vi "汇总各次拍照结果存档.vi"(8 "ModelEditInfo":T1={"Root"=path "", "AllModelFold"=path "", "AllModelNamePath"=path "", "所有零件型号"=[], "当前零件型号"="", "所有建立零件信息"=[], "当前零件序号"=0, "当前产品所有点位信息"={"当前点位序号"=0, "点位信息路径"=path "", "CAD点位坐标路径"=path "", "点位信息表"=[], "当前点位信息"={"点位名称"="", "点位坐标(图纸)"={"X"=0.0, "Y"=0.0, "Z"=0.0}, "点位坐标(实际)"={"X"=0.0, "Y"=0.0, "Z"=0.0, "R"=0.0}, "补偿值"={"X"=0.0, "Y"=0.0, "Z"=0.0}, "锁附时机械手角度"=enum."0度", "放料点相对于Mark\n拍照点高度差"=0.0, "选择螺丝托盘"=enum."托盘1", "拧紧程式序号"=0, "自动锁螺丝"=FALSE}, "CAD图纸点位个数"=0}, "当前产品信息"={"产品型号"="J016-9STWH-A插头", "螺丝刀型号"=enum."螺丝刀5-2.5*4mm", "载具上放几片PCB"=0, "1片PCB锁几颗螺丝"=0, "CAD点位坐标文档路径"=path "", "托盘1螺丝型号"=enum."十字螺丝M5*12", "托盘2螺丝型号"=enum."十字螺丝M5*12", "托盘3螺丝型号"=enum."不供料", "托盘4螺丝型号"=enum."不供料", "托盘5螺丝型号"=enum."一字螺丝M2.5*8", "托盘6螺丝型号"=enum."一字螺丝M2.5*8", "托盘7螺丝型号"=enum."一字螺丝M2.5*8", "托盘8螺丝型号"=enum."一字螺丝M2.5*8", "托盘1螺丝锁紧程式序号"=1, "托盘2螺丝锁紧程式序号"=0, "托盘3螺丝锁紧程式序号"=0, "托盘4螺丝锁紧程式序号"=0, "托盘5螺丝锁紧程式序号"=0, "托盘6螺丝锁紧程式序号"=0, "托盘7螺丝锁紧程式序号"=0, "托盘8螺丝锁紧程式序号"=0, "预锁程式序号"=0, "复锁程式序号"=0, "上相机拍PCB孔曝光时间"=0, "上相机取料拍螺帽曝光时间"=0, "上相机复锁拍螺帽曝光时间"=0, "下相机曝光时间"=0}, "所有螺丝和垫片型号"=[], "所有螺丝和垫片型号Path"=path "", "Mark拍照点坐标"=[], "自动锁螺丝: PCB孔拍照点坐标-多片PCB(去除未勾选的)"=[], "8个供料盘是否供料-1PCB(去除未勾选的)"=[], "8个供料盘是否拍照取料"=[], "自动锁螺丝: 1PCB每颗螺丝来自哪个供料盘U8(去除未勾选的)"=[], "自动锁螺丝: 1PCB每颗螺丝拧紧程式编号U8(去除未勾选的)"=[], "4个预锁程式+4个复锁程式编号U8"=[], "自动锁螺丝: 锁螺丝相对拍照时旋转角度-多片PCB(去除未勾选的)"=[], "自动锁螺丝: 点位补偿值-多片PCB(去除未勾选的)"=[], "1PCB上自动锁螺丝个数(去除未勾选的)"=0, "自动锁螺丝: 放料点相对拍照点高度差-多片PCB(去除未勾选的)"=[], "8个供料盘是否供料(包括未勾选的)"=[], "已勾选的自动锁螺丝点位供料盘设定错误"=FALSE} {"当前产品信息"."载具上放几片PCB" min=1 max=4; "当前产品信息"."托盘8螺丝锁紧程式序号" min=1 max=150 step=1; "当前产品信息"."托盘7螺丝锁紧程式序号" min=1 max=150 step=1; "当前产品信息"."托盘6螺丝锁紧程式序号" min=1 max=150 step=1; "当前产品信息"."托盘5螺丝锁紧程式序号" min=1 max=150 step=1; "当前产品信息"."复锁程式序号" min=1 max=150 step=1; "当前产品信息"."预锁程式序号" min=1 max=150 step=1; "当前产品信息"."托盘4螺丝锁紧程式序号" min=1 max=150 step=1; "当前产品信息"."托盘3螺丝锁紧程式序号" min=1 max=150 step=1; "当前产品信息"."托盘2螺丝锁紧程式序号" min=1 max=150 step=1; "当前产品信息"."托盘1螺丝锁紧程式序号" min=1 max=150 step=1; "当前产品所有点位信息"."当前点位信息"."放料点相对于Mark\n拍照点高度差" format="%.3g"}, 9 "不同产品总结果":bool[](array[boolean]), 11 "缓存待存储数据输入":T10) -> (0 "每个数据结果":bool[][](array[boolean]), 1 "数据":string[][](array[string]), 3 "存档数据为空":bool)   [LabVIEW 2014]
uses:
  ModelEditSubVIs/ModeEditeControl.ctl
  Controls/XYZPos.ctl
  Controls/XYZRPos.ctl
  ModelEditSubVIs/ModelInfo.ctl
  Global.vi
panel:
  out "波形图 2":dbl[][](graph)
  out "波形图":dbl[][](graph)
  # "mm   往下为正"
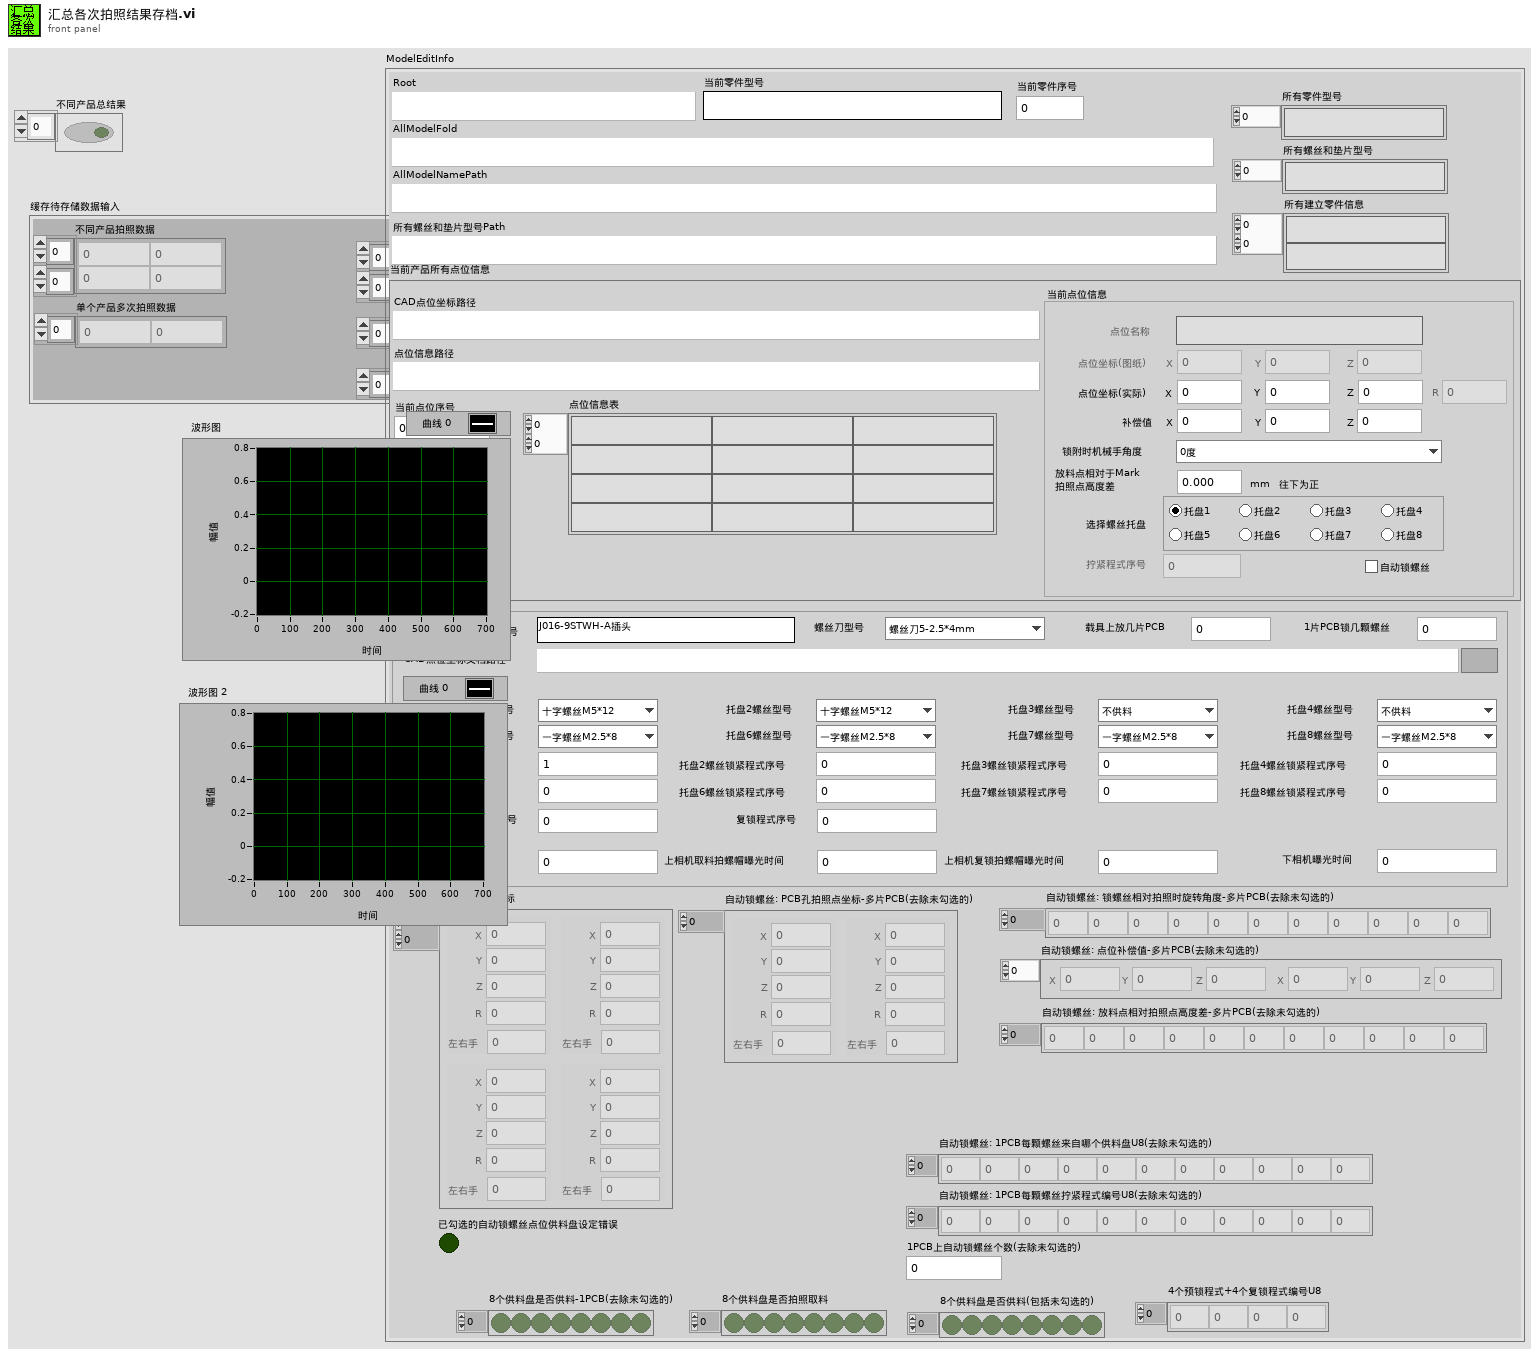
[diagram p1: front panel]
types:
  T1 = typedef "ModeEditeControl.ctl" = cluster{"Root":path, "AllModelFold":path, "AllModelNamePath":path, "所有零件型号":string[], "当前零件型号":string, "所有建立零件信息":string[][], "当前零件序号":i32, "当前产品所有点位信息":cluster{"当前点位序号":i32, "点位信息路径":path, "CAD点位坐标路径":path, "点位信息表":string[][], "当前点位信息":T2, "CAD图纸点位个数":i32}, "当前产品信息":T6, "所有螺丝和垫片型号":string[], "所有螺丝和垫片型号Path":path, "Mark拍照点坐标":T9[][], "自动锁螺丝: PCB孔拍照点坐标-多片PCB(去除未勾选的)":T9[], "8个供料盘是否供料-1PCB(去除未勾选的)":bool[], "8个供料盘是否拍照取料":bool[], "自动锁螺丝: 1PCB每颗螺丝来自哪个供料盘U8(去除未勾选的)":u8[], "自动锁螺丝: 1PCB每颗螺丝拧紧程式编号U8(去除未勾选的)":u8[], "4个预锁程式+4个复锁程式编号U8":u8[], "自动锁螺丝: 锁螺丝相对拍照时旋转角度-多片PCB(去除未勾选的)":i32[], "自动锁螺丝: 点位补偿值-多片PCB(去除未勾选的)":T3[], "1PCB上自动锁螺丝个数(去除未勾选的)":i32, "自动锁螺丝: 放料点相对拍照点高度差-多片PCB(去除未勾选的)":dbl[], "8个供料盘是否供料(包括未勾选的)":bool[], "已勾选的自动锁螺丝点位供料盘设定错误":bool}
  T2 = typedef "锁附点位信息.ctl" = cluster{"点位名称":string, "点位坐标(图纸)":T3, "点位坐标(实际)":T4, "补偿值":T3, "锁附时机械手角度":T5, "放料点相对于Mark\n拍照点高度差":dbl, "选择螺丝托盘":enum32{"托盘1", "托盘2", "托盘3", "托盘4", "托盘5", "托盘6", "托盘7", "托盘8"}, "拧紧程式序号":u16, "自动锁螺丝":bool}
  T3 = typedef "XYZPos.ctl" = cluster{"X":dbl, "Y":dbl, "Z":dbl}
  T4 = typedef "XYZRPos.ctl" = cluster{"X":dbl, "Y":dbl, "Z":dbl, "R":dbl}
  T5 = typedef "锁附时机械手角度.ctl" = enum16{"0度", "顺时针90度", "顺时针180度", "逆时针90度", "逆时针180度"}
  T6 = typedef "ModelInfo.ctl" = cluster{"产品型号":string, "螺丝刀型号":T7, "载具上放几片PCB":u16, "1片PCB锁几颗螺丝":u16, "CAD点位坐标文档路径":path, "托盘1螺丝型号":T8, "托盘2螺丝型号":T8, "托盘3螺丝型号":T8, "托盘4螺丝型号":T8, "托盘5螺丝型号":T8, "托盘6螺丝型号":T8, "托盘7螺丝型号":T8, "托盘8螺丝型号":T8, "托盘1螺丝锁紧程式序号":u32, "托盘2螺丝锁紧程式序号":u32, "托盘3螺丝锁紧程式序号":u32, "托盘4螺丝锁紧程式序号":u32, "托盘5螺丝锁紧程式序号":u32, "托盘6螺丝锁紧程式序号":u32, "托盘7螺丝锁紧程式序号":u32, "托盘8螺丝锁紧程式序号":u32, "预锁程式序号":u32, "复锁程式序号":u32, "上相机拍PCB孔曝光时间":u32, "上相机取料拍螺帽曝光时间":u32, "上相机复锁拍螺帽曝光时间":u32, "下相机曝光时间":u32}
  T7 = typedef "螺丝刀类型.ctl" = enum16{"螺丝刀1-1*3mm", "螺丝刀2-1.5*3mm", "螺丝刀3-2*3mm", "螺丝刀4-2*4mm", "螺丝刀5-2.5*4mm"}
  T8 = typedef "控件-螺丝型号.ctl" = enum16{"不供料", "一字螺丝M2.5*8", "一字螺丝M3*10", "一字螺丝M5*8", "一字螺丝M5*12", "十字螺丝M3*8", "十字螺丝M3*12", "十字螺丝M5*8", "十字螺丝M5*12"}
  T9 = typedef "XYZRPos+左右手.ctl" = cluster{"坐标":T4, "左右手":dbl}
  T10 = typedef "控件-缓存数据.ctl" = cluster{"不同产品拍照数据":dbl[][], "不同产品拍照结果":bool[][], "单个产品多次拍照数据":dbl[], "单个产品多次拍照结果":bool[], "不同产品总结果":bool[]}
  T11 = cluster{"不同产品拍照数据":dbl[], "不同产品拍照结果":bool[], "布尔":bool, bool}
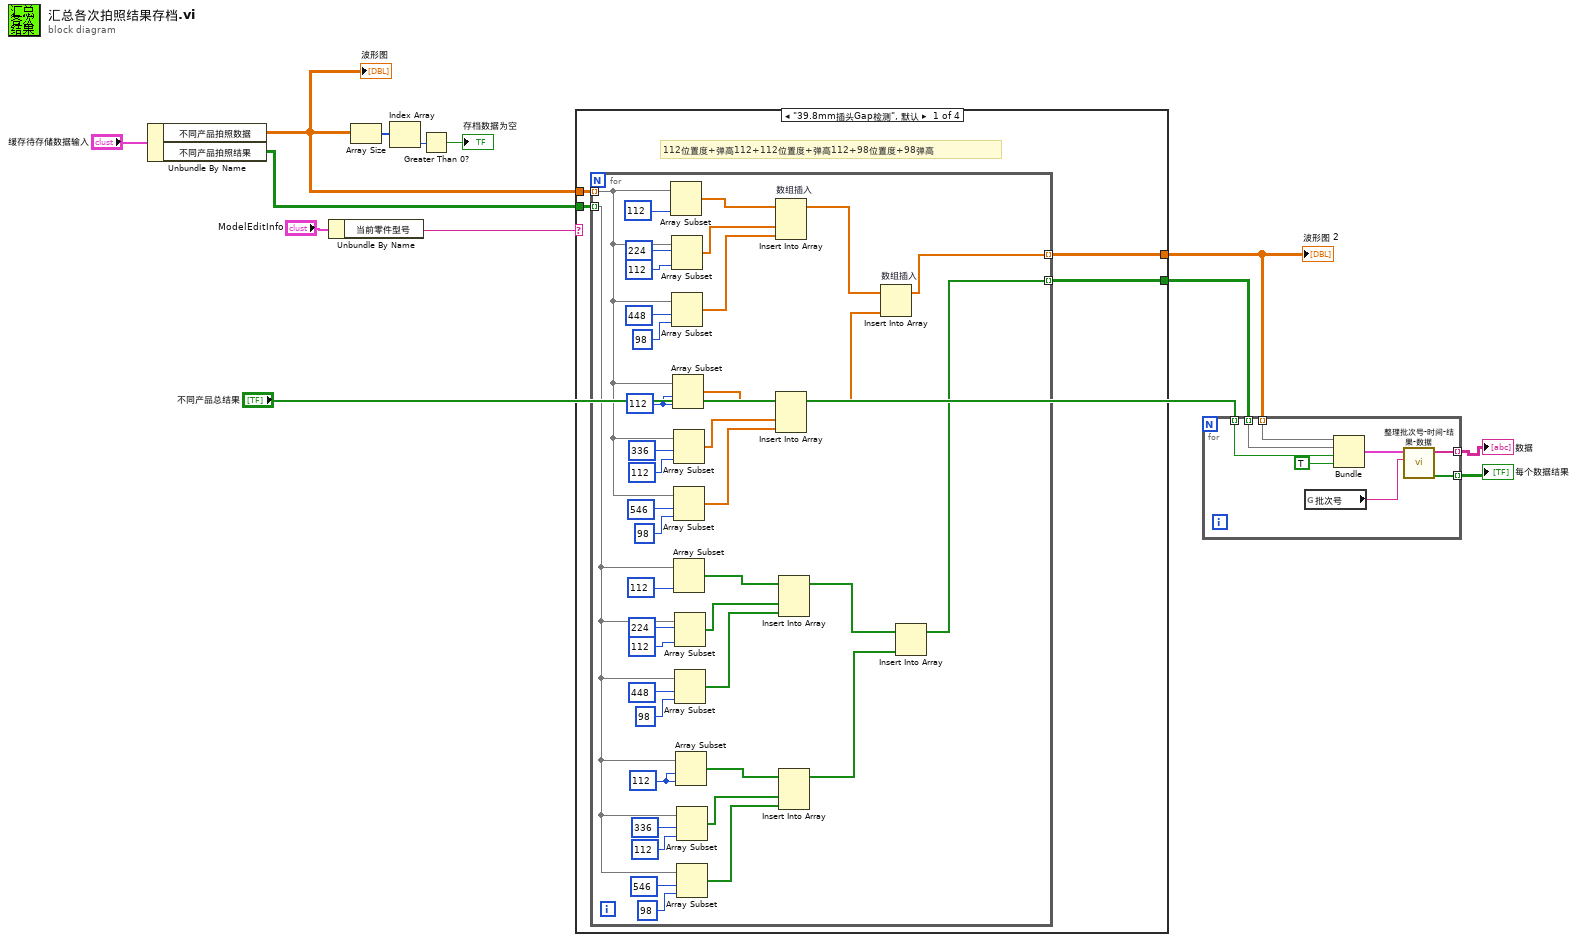
[diagram p0: block diagram]
diagram:
  n1 = Unbundle By Name("缓存待存储数据输入") -> ("不同产品拍照数据"=w6:dbl[][], "不同产品拍照结果"=w5:bool[][])
  "波形图" <- w6
  n2 = Unbundle By Name("ModelEditInfo") -> ("当前零件型号"=w8:string)
  n3 = Array Size(array=w6) -> (size(s)=w11:i32[])
  n4 = Index Array(array=w11) -> (element=w12:i32)  [unwired: 1 in]
  n5 = Greater Than 0?(x=w12) -> (x > 0?=→"存档数据为空":bool)
  n6 = case shown="\"39.8mm插头Gap检测\", 默认" w8 {
    tunnel: w6 -> [w17 w59 w61 w63]
    tunnel: w5 -> [w16 w58 w60 w62]
    tunnel: [w14 w59 w61 w63] -> w1
    tunnel: [w15 w58 w60 w62] -> w2
    frame "39.8mm插头Gap检测", Default {
      # "112位置度+弹高112+112位置度+弹高112+98位置度+98弹高"
      n7 = for {
        tunnel: w17 -> [w44] mode=indexing
        tunnel: w16 -> [w23] mode=indexing
        tunnel: [w22] -> w15 mode=indexing
        tunnel: [w18] -> w14 mode=indexing
        w39 = 112 ("长度")
        w43 = 112 ("长度")
        n8 = Array Subset(array=w44, length=112 ("长度")) -> (w19:dbl[])  [unwired: 1 in]
        n9 = Array Subset(array=w44, index=224 ("长度"), length=112 ("长度")) -> (w52:dbl[])
        n10 = Array Subset(array=w44, index=448 ("长度"), length=98 ("长度")) -> (w20:dbl[])
        n11 = Array Subset(array=w44, index=w43, length=w43) -> (w49:dbl[])
        n12 = Array Subset(array=w44, index=336 ("长度"), length=112 ("长度")) -> (w50:dbl[])
        n13 = Array Subset(array=w44, index=546 ("长度"), length=98 ("长度")) -> (w51:dbl[])
        n14 = Array Subset(array=w23, length=112 ("长度")) -> (w29:bool[])  [unwired: 1 in]
        n15 = Array Subset(array=w23, index=224 ("长度"), length=112 ("长度")) -> (w30:bool[])
        n16 = Array Subset(array=w23, index=448 ("长度"), length=98 ("长度")) -> (w31:bool[])
        n17 = Array Subset(array=w23, index=w39, length=w39) -> (w34:bool[])
        n18 = Array Subset(array=w23, index=336 ("长度"), length=112 ("长度")) -> (w33:bool[])
        n19 = Array Subset(array=w23, index=546 ("长度"), length=98 ("长度")) -> (w32:bool[])
        n20 = Insert Into Array "数组插入"(array=w19, new element #1=w52, new element #2=w20) -> (w21:dbl[])  [unwired: 1 in]
        n21 = Insert Into Array(array=w49, new element #1=w50, new element #2=w51) -> (w42:dbl[])  [unwired: 1 in]
        n22 = Insert Into Array(array=w29, new element #1=w30, new element #2=w31) -> (w40:bool[])  [unwired: 1 in]
        n23 = Insert Into Array(array=w34, new element #1=w33, new element #2=w32) -> (w41:bool[])  [unwired: 1 in]
        n24 = Insert Into Array "数组插入"(array=w21, new element=w42) -> (w18:dbl[])  [unwired: 1 in]
        n25 = Insert Into Array(array=w40, new element=w41) -> (w22:bool[])  [unwired: 1 in]
      }
    }
    frame "诺基亚检测" {
    }
    frame "39.8mm插头Gap检测校验" {
    }
    frame "诺基亚检测校验" {
    }
  }
  "波形图 2" <- w1
  n26 = for {
    tunnel: w1 -> [w71] mode=indexing
    tunnel: w2 -> [w70] mode=indexing
    tunnel: [w67] -> w4 mode=indexing
    tunnel: [w66] -> w3 mode=indexing
    tunnel: "不同产品总结果" -> [w65] mode=indexing
    n27 = global read "Global.vi" "批次号"() -> (w64:string)
    n28 = Bundle("不同产品拍照数据"=w71, "不同产品拍照结果"=w70, "布尔"=w65, TRUE) -> (w68:T11)  [unwired: 1 in]
    n29 = call "整理批次号-时间-结果-数据.vi"("批次号"=w64, "存档数据和结果"=w68) -> ("添加了批次号时间，结果的存档颜色"=w66:bool[], "数组"=w67:string[])  [unwired: 8 in]
  }
  "数据" <- w4
  "每个数据结果" <- w3
